vi "MonoTest.vi"() -> ()   [LabVIEW 2009]
panel:
  out "Busy":bool
  out "Response":string
  out "Command Complete":string
  in  "Exit":bool
  out "Read Error?":bool
  in  "Scan Speed (nm/min)":dbl=100.0 min=1.0 max=500.0 step=0.1 format="%.1f"
  in  "Wavelength (nm)":dbl=100.0 min=0.0 max=2000.0 step=0.1 format="%.1f"
  in  "Command":u16(ring) items=["nm", "goto", "nm/min", "VIS grating", "IR grating"]
  in  "Send Command":bool
  in  "Send Question":bool
  in  "Ask?":u16(ring) items=["?nm", "?nm/min", "?grating", "?turret", "?gratings"]
  in  "Mono Port":refnum<visa-resource-name>="COM5"
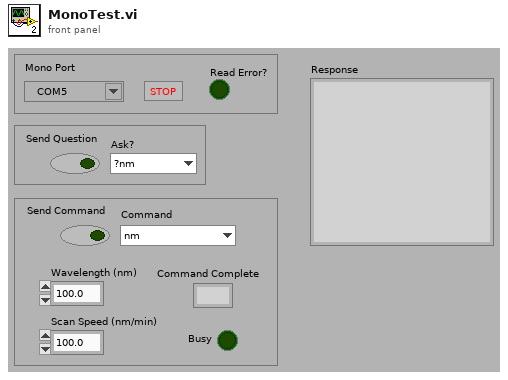
[diagram p1: front panel]
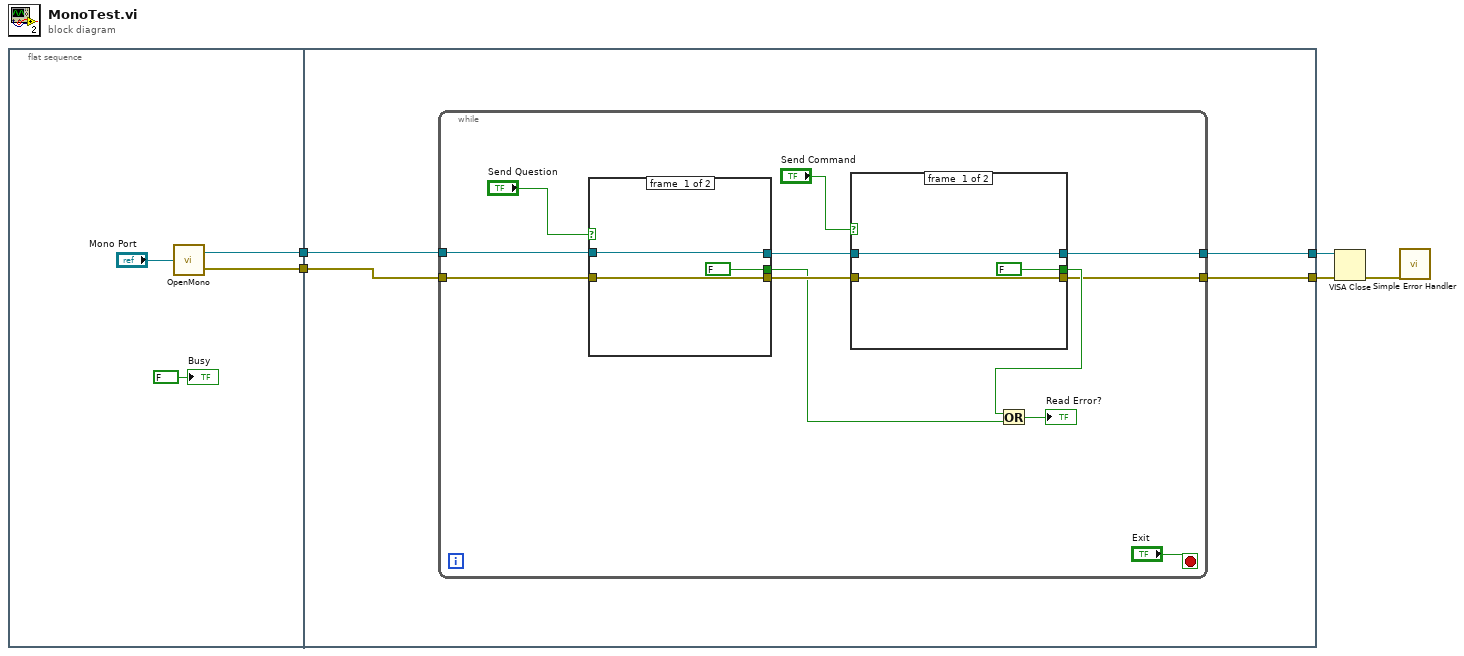
[diagram p0: block diagram]
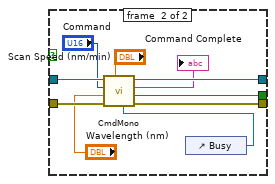
[diagram p2: hidden frame]
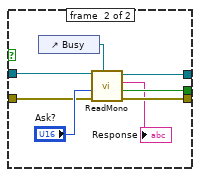
[diagram p3: hidden frame]
diagram:
  n1 = flat-sequence {
    tunnel: [w9] -> w5
    tunnel: [w8] -> w4
    tunnel: w5 -> [w13]
    tunnel: w4 -> [w12]
    tunnel: [w11] -> w2
    tunnel: [w10] -> w1
    frame #0 {
      n2 = call "OpenMono.vi"("Mono Port"="Mono Port") -> ("VISA resource name out"=w8:refnum<visa-resource-name>, "error out"=w9:errorcluster)
      "Busy" <- FALSE ("Busy")
    }
    frame #1 {
      n3 = while {
        tunnel: w13 -> [w22]
        tunnel: w12 -> [w23]
        tunnel: [w16] -> w11
        tunnel: [w15] -> w10
        stop <- "Exit" stop-if-true
        n4 = case shown="True" "Send Question" {
          tunnel: w23 -> [w41 w48]
          tunnel: w22 -> [w40 w47]
          tunnel: [w41 w46] -> w21
          tunnel: [w40 w45] -> w20
          tunnel: [FALSE ("Read Error") w44] -> w17
          frame #0 {
          }
          frame #1 {
            n5 = control-ref of="Busy"() -> (w42:refnum<vi>)
            n6 = call "ReadMono.vi"("Busy"=w42, "error in (no error)"=w47, "Cmd"="Ask?", "Mono Port"=w48) -> ("error out"=w45:errorcluster, "Read Error"=w44:bool, "Response"=→"Response":string, "Mono Port Out"=w46:refnum<visa-resource-name>)  [unwired: 2 in]
          }
        }
        n7 = case shown="True" "Send Command" {
          tunnel: w21 -> [w28 w38]
          tunnel: w20 -> [w27 w37]
          tunnel: [w28 w36] -> w16
          tunnel: [w27 w35] -> w15
          tunnel: [FALSE ("Read Error") w31] -> w18
          frame #0 {
          }
          frame #1 {
            n8 = control-ref of="Busy"() -> (w29:refnum<vi>)
            n9 = call "CmdMono.vi"("Busy"=w29, "Scan Speed (nm/min)"="Scan Speed (nm/min)", "error in (no error)"=w37, "Wavelength (nm)"="Wavelength (nm)", "Cmd"="Command", "Mono Port"=w38) -> ("error out"=w35:errorcluster, "Read Error"=w31:bool, "Response"=→"Command Complete":string, "Mono Port Out"=w36:refnum<visa-resource-name>)  [unwired: 2 in]
          }
        }
        n10 = Or(x=w18, y=w17) -> (x .or. y?=→"Read Error?":bool)
      }
    }
  }
  n11 = VISA Close(VISA resource name=w2, error in (no error)=w1) -> (error out=w3:errorcluster)
  n12 = call <vilib>:"Simple Error Handler.vi"("error in (no error)"=w3) -> ()  [unwired: 1 in, 8 out]
